vi "addStringElement.vi"(7 "Name":string, 8 "error in (no error)":errorcluster, 9 "Value":string, 10 "Replace? (false)":bool, 11 "tBSONDocument in":refnum<class "tBSONDocument.lvclass">) -> (0 "error out":errorcluster, 3 "tBSONDocument out":refnum<class "tBSONDocument.lvclass">)   [LabVIEW 2013, in "BSON.lvlib" / "tBSONDocument.lvclass"]
doc: "Adds a string to a BSON document."
uses:
  tBSONDocument.lvclass
  BSONElements/tBSONString/tBSONString.lvclass
  tBSONElement/tBSONElement.lvclass
  tBSONElement/setName.vi
  BSONElements/tBSONString/setValue.vi
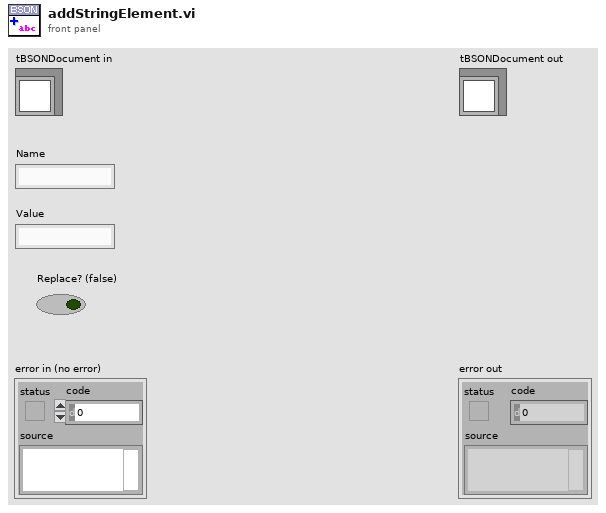
[diagram p1: front panel]
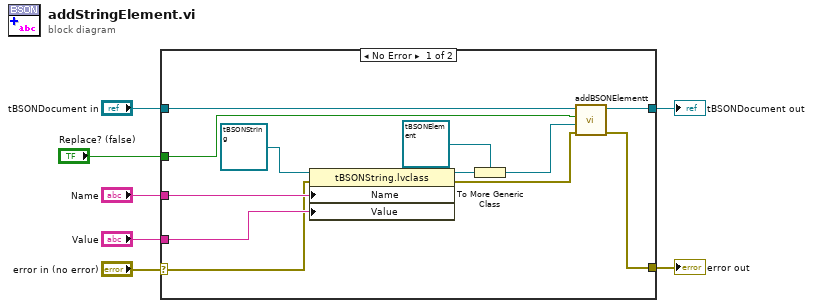
[diagram p0: block diagram]
diagram:
  n1 = case shown="No Error" "error in (no error)" {
    selector: "error in (no error)" -> [w13 w21]
    tunnel: [w18 w21] -> w6
    tunnel: [w19 w20] -> w4
    tunnel: "tBSONDocument in" -> [w14 w20]
    tunnel: "Name" -> [w15 _]
    tunnel: "Value" -> [w17 _]
    tunnel: "Replace? (false)" -> [w8 _]
    frame No Error {
      n2 = property class="tBSONString.lvclass"(reference=refnum<class "tBSONString.lvclass"> refnum ("BSON.lvlib:tBSONString.lvclass"), error in=w13, "Name"=w15, "Value"=w17) -> (reference out=w12:refnum<class "tBSONString.lvclass">, error out=w10:errorcluster)
      n3 = To More Generic Class(target class=refnum<class "tBSONElement.lvclass"> refnum ("BSON.lvlib:tBSONElement.lvclass"), reference=w12) -> (generic class reference=w9:refnum<class "tBSONElement.lvclass">)
      n4 = call "addBSONElementt.vi"("error in (no error)"=w10, "Element"=w9, "Replace? (false)"=w8, "tBSONDocument in"=w14) -> ("error out"=w18:errorcluster, "tBSONDocument out"=w19:refnum<class "tBSONDocument.lvclass">)  [unwired: 6 in]
    }
    frame Error {
    }
  }
  "error out" <- w6
  "tBSONDocument out" <- w4
